vi "Pre Launch Init.vi"(11 "SpectrometerUI in":refnum<class "SpectrometerUI.lvclass">) -> (0 "error out":errorcluster, 3 "SpectrometerUI out":refnum<class "SpectrometerUI.lvclass">)   [LabVIEW 2023, in "SpectrometerUI.lvlib" / "SpectrometerUI.lvclass"]
doc: "(<B>Filename</B>: Actor Framework.lvlib:Actor.lvclass:Pre Launch Init.vi)\n\nDefines behavior that occurs after the Launch Nested Actor method is invoked but before the actor's Actor Core method begins running.\n\nBy default, this method does nothing. A descendant class may override it to define behavior."
uses:
  SpectrometerUI.lvclass
  SpectrometerUI.lvclass/SpectrometerUI.ctl
  <vilib>/ActorFramework/Actor/Actor.lvclass
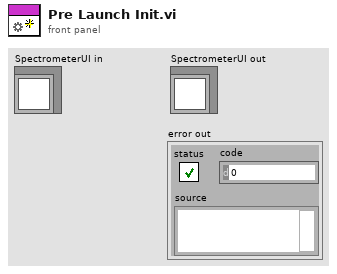
[diagram p1: front panel]
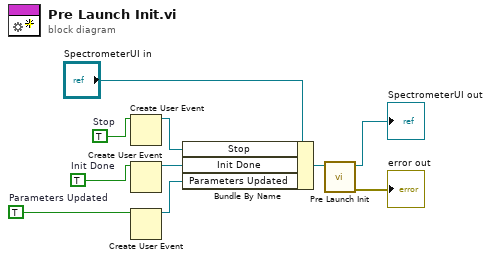
[diagram p0: block diagram]
diagram:
  w3 = TRUE  # Parameters Updated
  w4 = TRUE  # Init Done
  w8 = TRUE  # Stop
  n1 = Create User Event(user event datatype=w8) -> (user event=w7:refnum<user-event>)  [unwired: 1 in, 1 out]
  n2 = Create User Event(user event datatype=w4) -> (user event=w2:refnum<user-event>)  [unwired: 1 in, 1 out]
  n3 = Create User Event(user event datatype=w3) -> (user event=w1:refnum<user-event>)  [unwired: 1 in, 1 out]
  n4 = Bundle By Name(cluster="SpectrometerUI in", "Stop"=w7, "Init Done"=w2, "Parameters Updated"=w1) -> (w5:refnum<class "SpectrometerUI.lvclass">)
  n5 = call-parent "Pre Launch Init.vi"("Actor in"=w5) -> ("error out"=→"error out":errorcluster, "Actor out"=→"SpectrometerUI out":refnum<class "SpectrometerUI.lvclass">)  [unwired: 9 in]
